vi "SHIFTER.vi"() -> (8 "SHIFTER DATA":T1)   [LabVIEW 2015, in "TLB` Template.lvlib"]
doc: "TLB Prime - Application Template 1.3.0.24\nNorm Kirchner, NI Systems Engineering - NI\nCopyright (c) 2014, NI"
uses:
  TLB` Template.lvlib
  TypeDef - SHIFTER.ctl
  State Declaration.ctl
  Dependencies.llb/Exit Event Ref.ctl
  Dependencies.llb/TLB`_Dependencies.lvlib
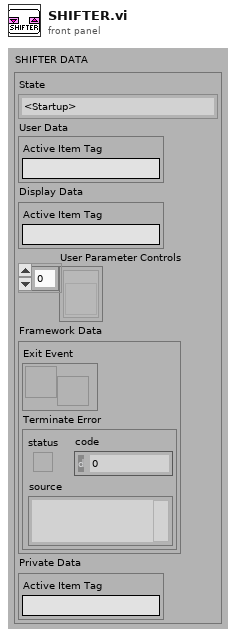
[diagram p1: front panel]
types:
  T1 = typedef "TLB` Template.lvlib/TypeDef - SHIFTER.ctl" = cluster{"State":T2, "User Data":cluster{"Active Item Tag":string}, "Display Data":cluster{"Active Item Tag":string}, "User Parameter Controls":refnum<vi>[], "Framework Data":cluster{"Exit Event":T3, "Terminate Error":errorcluster}, "Private Data":cluster{"Active Item Tag":string}}
  T2 = typedef "TLB` Template.lvlib/State Declaration.ctl" = enum16{"<Startup>", "Idle", "<Shutdown>"}
  T3 = typedef "TLB` Template.lvlib/TLB`_Dependencies.lvlib/Exit Event Ref.ctl" = refnum<user-event>
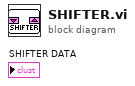
[diagram p0: block diagram]
diagram:
